vi "pressureSensor_Init.vi"(8 "error in (no error)":errorcluster, 11 "pressureSensor in":refnum<class "pressureSensor.lvclass">) -> (0 "error out":errorcluster, 3 "pressureSensor out":refnum<class "pressureSensor.lvclass">)   [LabVIEW 2020, in "RPI.SenseHat.Sensors.lvlib" / "pressureSensor.lvclass"]
uses:
  pressureSensor.lvclass
  pressureSensor.lvclass/pressureSensor.ctl
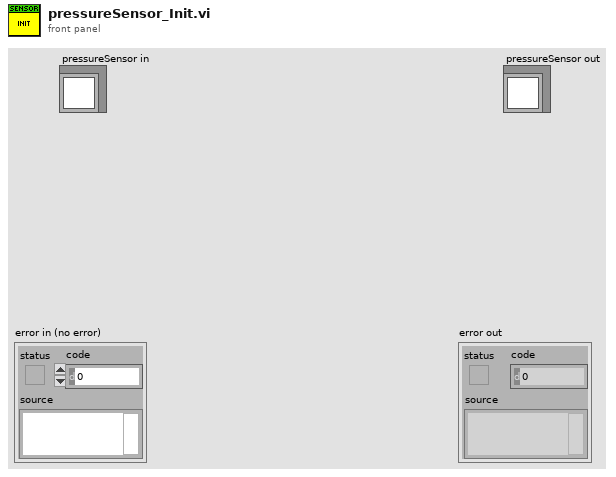
[diagram p1: front panel]
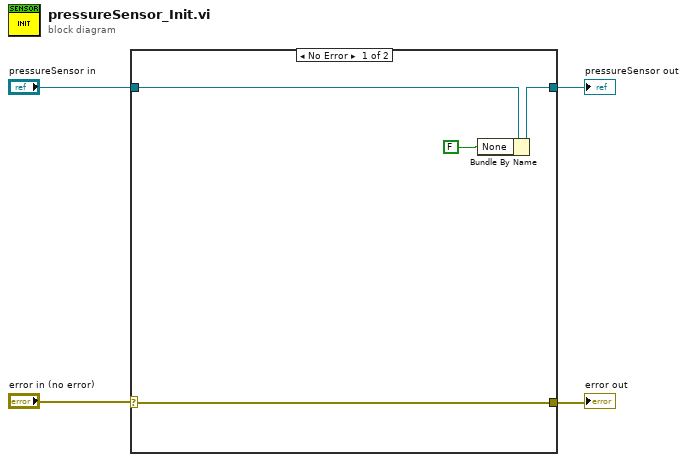
[diagram p0: block diagram]
diagram:
  n1 = case shown="No Error" "error in (no error)" {
    selector: "error in (no error)" -> [w5 w9]
    tunnel: "pressureSensor in" -> [w8 w10]
    tunnel: [w7 w10] -> w3
    tunnel: [w5 w9] -> w1
    frame No Error {
      n2 = Bundle By Name(cluster=w8, "None"=FALSE) -> (w7:refnum<class "pressureSensor.lvclass">)
    }
    frame Error {
    }
  }
  "pressureSensor out" <- w3
  "error out" <- w1
